vi "search_command_from_LUT_and_quiry.vi"(3 "parameter_string":string, 4 "input_general_command":string, 5 "input_machine_reference.lvclass":refnum<class "machine.lvclass">) -> (0 "quiry_result":string, 1 "output_specific_command":string, 2 "output_machine_reference.lvclass":refnum<class "machine.lvclass">)   [LabVIEW 2014, in "machine.lvclass"]
uses:
  machine.lvclass
  machine.lvclass/machine.ctl
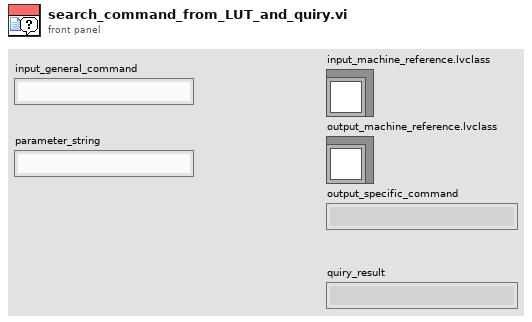
[diagram p1: front panel]
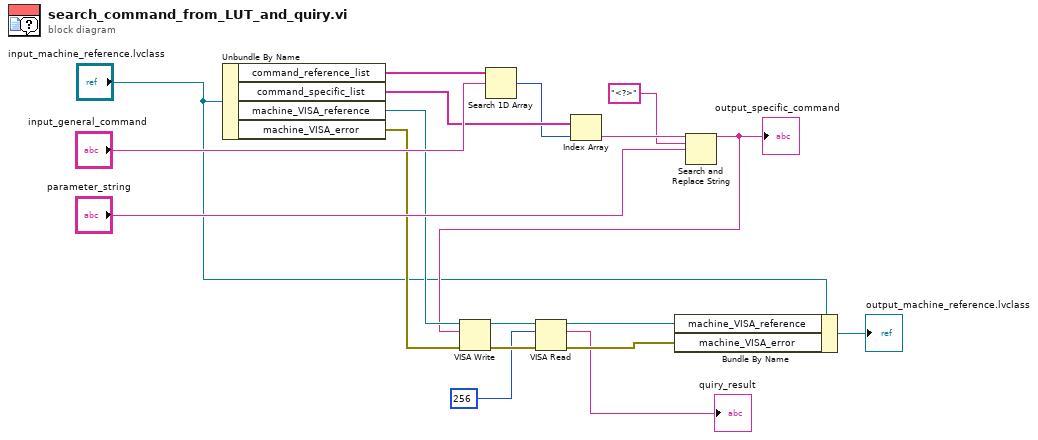
[diagram p0: block diagram]
diagram:
  n1 = Unbundle By Name("input_machine_reference.lvclass") -> ("command_reference_list"=w18:string[], "command_specific_list"=w16:string[], "machine_VISA_reference"=w11:refnum<visa-resource-name>, "machine_VISA_error"=w10:errorcluster)
  n2 = Search 1D Array(1D array=w18, element="input_general_command") -> (index of element=w15:i32)  [unwired: 1 in]
  n3 = Index Array(array=w16, index=w15) -> (element=w14:string)
  n4 = Search and Replace String(input string=w14, search string="<?>", replace string="parameter_string") -> (result string=w9:string)  [unwired: 5 in, 3 out]
  "output_specific_command" <- w9
  n5 = VISA Write(VISA resource name=w11, write buffer=w9, error in (no error)=w10) -> (VISA resource name out=w6:refnum<visa-resource-name>, error out=w5:errorcluster)  [unwired: 1 out]
  n6 = VISA Read(VISA resource name=w6, byte count=u32 256, error in (no error)=w5) -> (VISA resource name out=w3:refnum<visa-resource-name>, read buffer=→"quiry_result":string, error out=w2:errorcluster)  [unwired: 1 out]
  n7 = Bundle By Name(cluster="input_machine_reference.lvclass", "machine_VISA_reference"=w3, "machine_VISA_error"=w2) -> (→"output_machine_reference.lvclass":refnum<class "machine.lvclass">)
